vi "generate property tests.vi"(8 "error in (no error)":errorcluster, 11 "Tdms File":refnum<k34>) -> (0 "error out":errorcluster, 3 "Tdms File Out":refnum<k34>)   [LabVIEW 2020]
doc: "Writes alternating segments of 2 sets of channels in the same group. ch1-3 at 1000 per write and 4-6 at 500 per write.\n\nEach pair of writes is alternated between interleaved and decimated data."
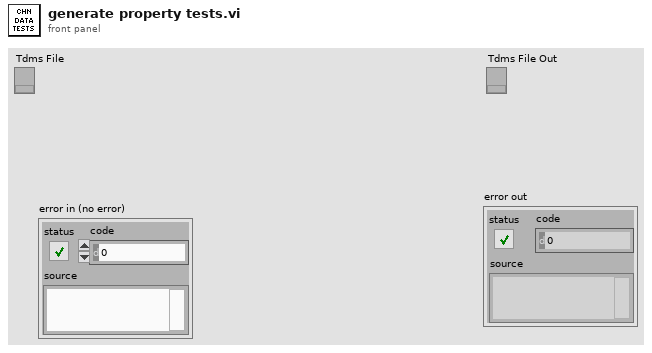
[diagram p1: front panel]
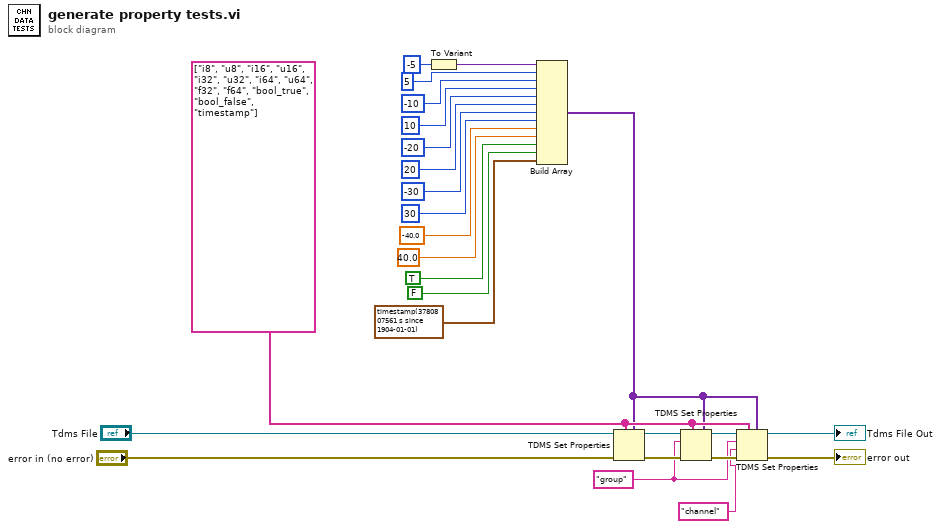
[diagram p0: block diagram]
diagram:
  w5 = "group" ("group name")
  w6 = string[] ["i8", "u8", "i16", "u16", "i32", "u32", "i64", "u64", "f32", "f64", "bool_true", "bool_false", "timestamp"]
  n1 = To Variant(anything=i8 -5) -> (Variant=w25:variant)
  n2 = Build Array(w25, u8 5, i16 -10, u8 10, -20, u32 20, i64 -30, u64 30, sgl -40.0, 40.0, TRUE, FALSE, timestamp(3780807561 s since 1904-01-01) ("Time Stamp")) -> (w1:variant[])
  n3 = TDMS Set Properties(5:w1, 7:w6, 8:"error in (no error)", 11:"Tdms File") -> (0:w9:errorcluster, 3:w10:refnum<k34>)  [unwired: 2 in, 2 out]
  n4 = TDMS Set Properties(5:w1, 7:w6, 8:w9, 10:w5, 11:w10) -> (0:w7:errorcluster, 3:w8:refnum<k34>)  [unwired: 1 in, 2 out]
  n5 = TDMS Set Properties(5:w1, 7:w6, 8:w7, 9:"channel" ("group name"), 10:w5, 11:w8) -> (0:→"error out":errorcluster, 3:→"Tdms File Out":refnum<k34>)  [unwired: 2 out]
